vi "AlliGator Check Fit Result Constraints.vi"(6 "Array of Decay Fit Result Constraints":T1[](array[typedef]), 7 "Max Relative Residual":dbl, 8 "Error In":errorcluster, 9 "Fit Parameters":dbl[](array[numeric]), 10 "ACF SDV":dbl, 11 "ACF Mean":dbl) -> (0 "Error Out":errorcluster, 3 "Constraints Stisfied?":bool)   [LabVIEW 2021, in "AlliGator Decay Fit Parameter Map.lvlib"]
doc: "Checks whether the fit parameters and derived quantities verify all the provided constraints."
uses:
  AlliGator Decay Fit Parameter Map.lvlib
  Fits/IRF(X)PSED/Decay Fit Result Constraint.ctl
  Fits/Fits.lvlib
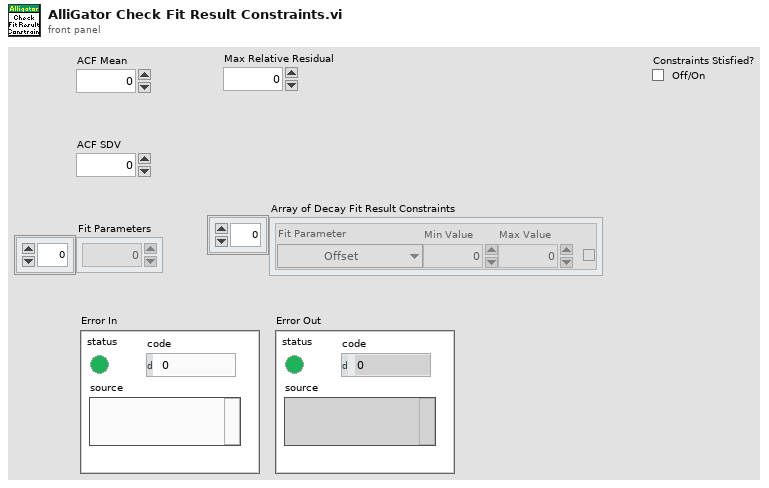
[diagram p1: front panel]
types:
  T1 = typedef "Fits.lvlib/Decay Fit Result Constraint.ctl" = cluster{"Fit Parameter":enum16{"Offset", "Baseline", "A_1", "tau_1", "A_2", "tau_2", "<tau>_a", "f1_a", "f2_a", "<tau>_i", "f1_i", "f2_i", "-", "R^2", "Chi^2", "Max Relative Residual", "<Residual ACF>", "Residual ACF SDV", "tau_2/tau_1"}, "Min Value":dbl, "Max Value":dbl, "Use Constraint":bool}
  T2 = enum16{"Offset", "Baseline", "A_1", "tau_1", "A_2", "tau_2", "<tau>_a", "f1_a", "f2_a", "<tau>_i", "f1_i", "f2_i", "-", "R^2", "Chi^2", "Max Relative Residual", "<Residual ACF>", "Residual ACF SDV", "tau_2/tau_1"}
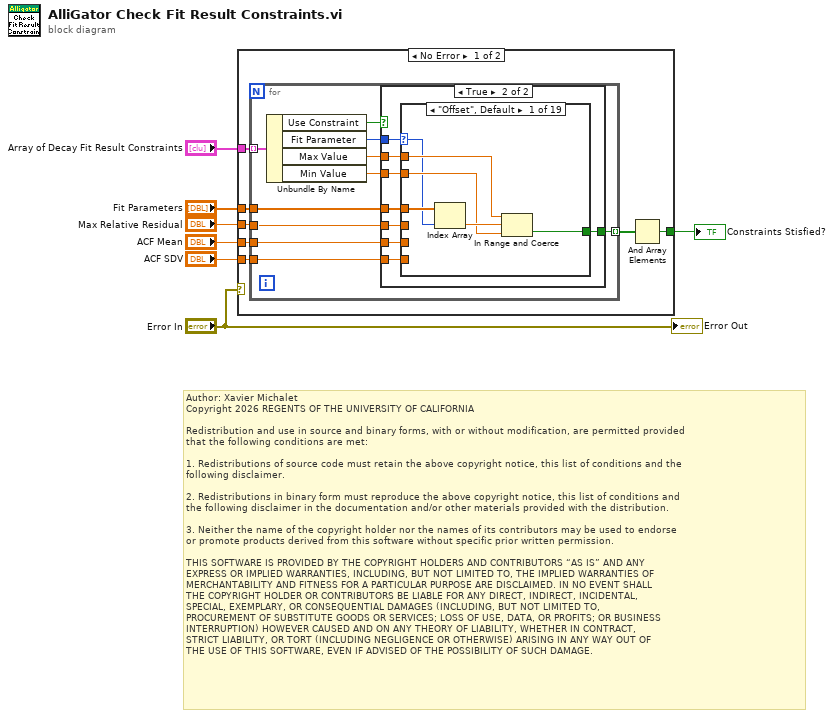
[diagram p0: block diagram]
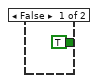
[diagram p2: hidden frame]
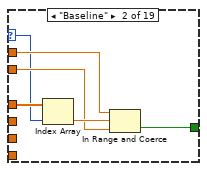
[diagram p3: hidden frame]
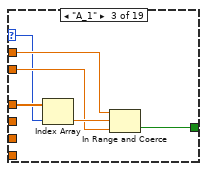
[diagram p4: hidden frame]
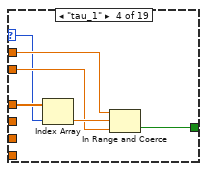
[diagram p5: hidden frame]
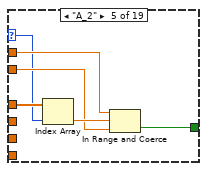
[diagram p6: hidden frame]
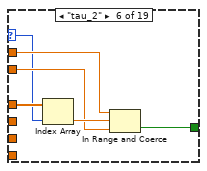
[diagram p7: hidden frame]
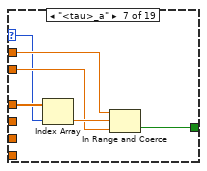
[diagram p8: hidden frame]
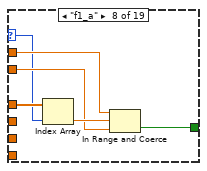
[diagram p9: hidden frame]
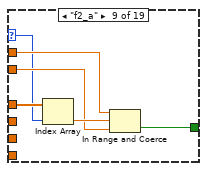
[diagram p10: hidden frame]
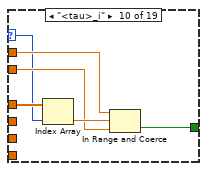
[diagram p11: hidden frame]
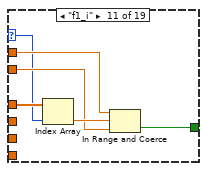
[diagram p12: hidden frame]
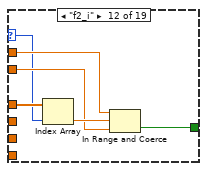
[diagram p13: hidden frame]
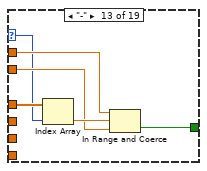
[diagram p14: hidden frame]
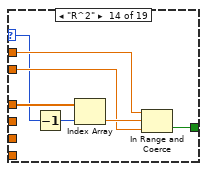
[diagram p15: hidden frame]
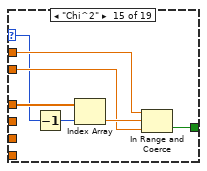
[diagram p16: hidden frame]
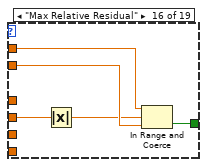
[diagram p17: hidden frame]
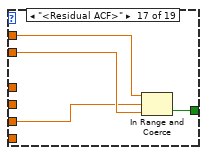
[diagram p18: hidden frame]
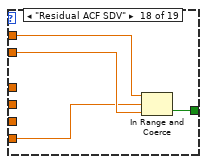
[diagram p19: hidden frame]
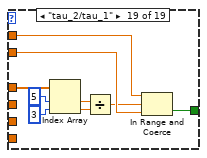
[diagram p20: hidden frame]
diagram:
  # "Author: Xavier Michalet\nCopyright 2026 REGENTS OF THE UNIVERSITY OF CALIFORNIA\n\nRedistribution and use in source and binary forms, with or without modification, are permitted provided\nthat the following conditions are met:\n\n1. Redistributions of source code must retain the above copyright notice, this list of conditions and the\nfollowing disclaimer.\n\n2. Redistributions in binary form must reproduce the above copyright notice, this list of conditions and\nthe following disclaimer in the documentation and/or other materials provided with the distribution.\n\n3. Neither the name of the copyright holder nor the names of its contributors may be used to endorse \nor promote products derived from this software without specific prior written permission.\n\nTHIS SOFTWARE IS PROVIDED BY THE COPYRIGHT HOLDERS AND CONTRIBUTORS “AS IS” AND ANY \nEXPRESS OR IMPLIED WARRANTIES, INCLUDING, BUT NOT LIMITED TO, THE IMPLIED WARRANTIES OF\nMERCHANTABILITY AND FITNESS FOR A PARTICULAR PURPOSE ARE DISCLAIMED. IN NO EVENT SHALL\nTHE COPYRIGHT HOLDER OR CONTRIBUTORS BE LIABLE FOR ANY DIRECT, INDIRECT, INCIDENTAL, \nSPECIAL, EXEMPLARY, OR CONSEQUENTIAL DAMAGES (INCLUDING, BUT NOT LIMITED TO, \nPROCUREMENT OF SUBSTITUTE GOODS OR SERVICES; LOSS OF USE, DATA, OR PROFITS; OR BUSINESS\nINTERRUPTION) HOWEVER CAUSED AND ON ANY THEORY OF LIABILITY, WHETHER IN CONTRACT, \nSTRICT LIABILITY, OR TORT (INCLUDING NEGLIGENCE OR OTHERWISE) ARISING IN ANY WAY OUT OF\nTHE USE OF THIS SOFTWARE, EVEN IF ADVISED OF THE POSSIBILITY OF SUCH DAMAGE."
  n1 = case shown="No Error" "Error In" {
    tunnel: "Array of Decay Fit Result Constraints" -> [w14 _]
    tunnel: "Fit Parameters" -> [w13 _]
    tunnel: "Max Relative Residual" -> [w12 _]
    tunnel: "ACF Mean" -> [w11 _]
    tunnel: "ACF SDV" -> [w10 _]
    tunnel: [w8 _] -> w1
    frame No Error {
      n2 = for {
        tunnel: w14 -> [w24] mode=indexing
        tunnel: w13 -> [w22]
        tunnel: [w18] -> w9 mode=indexing
        tunnel: w12 -> [w17]
        tunnel: w11 -> [w16]
        tunnel: w10 -> [w15]
        n3 = Unbundle By Name(w24) -> ("Use Constraint"=w21:bool, "Fit Parameter"=w23:T2, "Max Value"=w20:dbl, "Min Value"=w19:dbl)
        n4 = case shown="True" w21 {
          tunnel: w23 -> [_ w33]
          tunnel: w22 -> [_ w32]
          tunnel: w20 -> [_ w31]
          tunnel: w19 -> [_ w30]
          tunnel: [TRUE w29] -> w18
          tunnel: w17 -> [_ w28]
          tunnel: w16 -> [_ w27]
          tunnel: w15 -> [_ w26]
          frame False {
          }
          frame True {
            n5 = case shown="\"Offset\", Default" w33 {
              selector: w33 -> [w34 w40 w46 w52 w58 w64 w70 w76 w82 w88 w94 w100 w106 w113 w120 _ _ _ _]
              tunnel: w32 -> [w39 w45 w51 w57 w63 w69 w75 w81 w87 w93 w99 w105 w111 w118 w125 _ _ _ w144]
              tunnel: w31 -> [w37 w43 w49 w55 w61 w67 w73 w79 w85 w91 w97 w103 w109 w116 w123 w130 w134 w138 w147]
              tunnel: w30 -> [w36 w42 w48 w54 w60 w66 w72 w78 w84 w90 w96 w102 w108 w115 w122 w129 w133 w137 w146]
              tunnel: [w35 w41 w47 w53 w59 w65 w71 w77 w83 w89 w95 w101 w107 w114 w121 w128 w132 w136 w145] -> w29
              tunnel: w28 -> [_ _ _ _ _ _ _ _ _ _ _ _ _ _ _ w127 _ _ _]
              tunnel: w27 -> [_ _ _ _ _ _ _ _ _ _ _ _ _ _ _ _ w131 _ _]
              tunnel: w26 -> [_ _ _ _ _ _ _ _ _ _ _ _ _ _ _ _ _ w135 _]
              frame "Offset", Default {
                n6 = Index Array(array=w39, index=w34) -> (element=w38:dbl)
                n7 = In Range and Coerce(upper limit=w37, x=w38, lower limit=w36) -> (In Range?=w35:bool)  [unwired: 1 out]
              }
              frame "Baseline" {
                n8 = Index Array(array=w45, index=w40) -> (element=w44:dbl)
                n9 = In Range and Coerce(upper limit=w43, x=w44, lower limit=w42) -> (In Range?=w41:bool)  [unwired: 1 out]
              }
              frame "A_1" {
                n10 = Index Array(array=w51, index=w46) -> (element=w50:dbl)
                n11 = In Range and Coerce(upper limit=w49, x=w50, lower limit=w48) -> (In Range?=w47:bool)  [unwired: 1 out]
              }
              frame "tau_1" {
                n12 = Index Array(array=w57, index=w52) -> (element=w56:dbl)
                n13 = In Range and Coerce(upper limit=w55, x=w56, lower limit=w54) -> (In Range?=w53:bool)  [unwired: 1 out]
              }
              frame "A_2" {
                n14 = Index Array(array=w63, index=w58) -> (element=w62:dbl)
                n15 = In Range and Coerce(upper limit=w61, x=w62, lower limit=w60) -> (In Range?=w59:bool)  [unwired: 1 out]
              }
              frame "tau_2" {
                n16 = Index Array(array=w69, index=w64) -> (element=w68:dbl)
                n17 = In Range and Coerce(upper limit=w67, x=w68, lower limit=w66) -> (In Range?=w65:bool)  [unwired: 1 out]
              }
              frame "<tau>_a" {
                n18 = Index Array(array=w75, index=w70) -> (element=w74:dbl)
                n19 = In Range and Coerce(upper limit=w73, x=w74, lower limit=w72) -> (In Range?=w71:bool)  [unwired: 1 out]
              }
              frame "f1_a" {
                n20 = Index Array(array=w81, index=w76) -> (element=w80:dbl)
                n21 = In Range and Coerce(upper limit=w79, x=w80, lower limit=w78) -> (In Range?=w77:bool)  [unwired: 1 out]
              }
              frame "f2_a" {
                n22 = Index Array(array=w87, index=w82) -> (element=w86:dbl)
                n23 = In Range and Coerce(upper limit=w85, x=w86, lower limit=w84) -> (In Range?=w83:bool)  [unwired: 1 out]
              }
              frame "<tau>_i" {
                n24 = Index Array(array=w93, index=w88) -> (element=w92:dbl)
                n25 = In Range and Coerce(upper limit=w91, x=w92, lower limit=w90) -> (In Range?=w89:bool)  [unwired: 1 out]
              }
              frame "f1_i" {
                n26 = Index Array(array=w99, index=w94) -> (element=w98:dbl)
                n27 = In Range and Coerce(upper limit=w97, x=w98, lower limit=w96) -> (In Range?=w95:bool)  [unwired: 1 out]
              }
              frame "f2_i" {
                n28 = Index Array(array=w105, index=w100) -> (element=w104:dbl)
                n29 = In Range and Coerce(upper limit=w103, x=w104, lower limit=w102) -> (In Range?=w101:bool)  [unwired: 1 out]
              }
              frame "-" {
                n30 = Index Array(array=w111, index=w106) -> (element=w110:dbl)
                n31 = In Range and Coerce(upper limit=w109, x=w110, lower limit=w108) -> (In Range?=w107:bool)  [unwired: 1 out]
              }
              frame "R^2" {
                n32 = Decrement(x=w113) -> (x-1=w112:T2)
                n33 = Index Array(array=w118, index=w112) -> (element=w117:dbl)
                n34 = In Range and Coerce(upper limit=w116, x=w117, lower limit=w115) -> (In Range?=w114:bool)  [unwired: 1 out]
              }
              frame "Chi^2" {
                n35 = Decrement(x=w120) -> (x-1=w119:T2)
                n36 = Index Array(array=w125, index=w119) -> (element=w124:dbl)
                n37 = In Range and Coerce(upper limit=w123, x=w124, lower limit=w122) -> (In Range?=w121:bool)  [unwired: 1 out]
              }
              frame "Max Relative Residual" {
                n38 = Absolute Value(x=w127) -> (abs(x)=w126:dbl)
                n39 = In Range and Coerce(upper limit=w130, x=w126, lower limit=w129) -> (In Range?=w128:bool)  [unwired: 1 out]
              }
              frame "<Residual ACF>" {
                n40 = In Range and Coerce(upper limit=w134, x=w131, lower limit=w133) -> (In Range?=w132:bool)  [unwired: 1 out]
              }
              frame "Residual ACF SDV" {
                n41 = In Range and Coerce(upper limit=w138, x=w135, lower limit=w137) -> (In Range?=w136:bool)  [unwired: 1 out]
              }
              frame "tau_2/tau_1" {
                n42 = Index Array(array=w144, index #1=5 ("index"), index #2=3 ("index")) -> (element #1=w141:dbl, element #2=w140:dbl)
                n43 = Divide(x=w141, y=w140) -> (x/y=w139:dbl)
                n44 = In Range and Coerce(upper limit=w147, x=w139, lower limit=w146) -> (In Range?=w145:bool)  [unwired: 1 out]
              }
            }
          }
        }
      }
      n45 = And Array Elements(Boolean array=w9) -> (logical AND=w8:bool)
    }
    frame Error {
    }
  }
  "Constraints Stisfied?" <- w1
  "Error Out" <- "Error In"
